vi "Sandbox.vi"() -> ()   [LabVIEW 2019, in "SV_Publisher.lvclass"]
uses:
  SV_Publisher.lvclass
  TypeDef/Needle Valve Data.ctl
  modbus engine custom/MB_ENGINE_class/Engine State.ctl
  TypeDef/Needle Valve State.ctl
  modbus engine custom/MB_ENGINE_class/Engine Alarms.ctl
  modbus engine custom/MB_ENGINE_class/Settings.ctl
  modbus engine custom/MB_ENGINE_class/Limits Status.ctl
  SV_Publisher.lvclass/SV_Publisher.ctl
  Set SV.vi/1ae5d02c-efd0-450a-8aa4-8388e25d05bc.vi
  modbus engine custom/MB_ENGINE_class/MB_ENGINE.lvclass
panel:
  in  "?":T1={"Engine State"=8, "StateValveModbus"=enum."IDLE", "Alarms"={"OL"=FALSE, "TF"=FALSE, "STL"=FALSE, "OCP"=FALSE, "CPUV"=FALSE, "UVLO"=FALSE, "SPI_ERROR"=FALSE, "Fault"=FALSE, "OL 2"=FALSE, "TF 2"=FALSE, "STL 2"=FALSE, "OCP 2"=FALSE, "CPUV 2"=FALSE, "UVLO 2"=FALSE, "reserved"=TRUE, "InitDone"=TRUE}, "RAW Possition"=124110, "Angele"=0.0, "Step"=0, "Encoder"=0, "Kinematic"={"ACC Steps Per Sec^2"=100, "DEC Steps Per Sec^2"=100, "Min Velosity Step Per Sec"=100, "Max Velosity Step Per Sec"=200, "MicroStep"=16}, "Limits"={"Fault 2 Switch"=FALSE, "Fault 1 Switch"=FALSE, "Center(Home)"=FALSE, "Lower Limit"=FALSE, "Upper Limit"=FALSE}} {"Engine State" items=["ACCELERATING", "DECELERATINGTOSTOP", "DECELERATING", "STEADY", "INDEX_ACCEL", "NDEX_RUN", "INDEX_DECEL", "INDEX_DWELL", "INACTIVE", "STANDBY", "STANDBYTOINACTIVE"]}
  in  "set 2":bool
  in  "set 1":bool
  in  "stop":bool
  out "error out":errorcluster
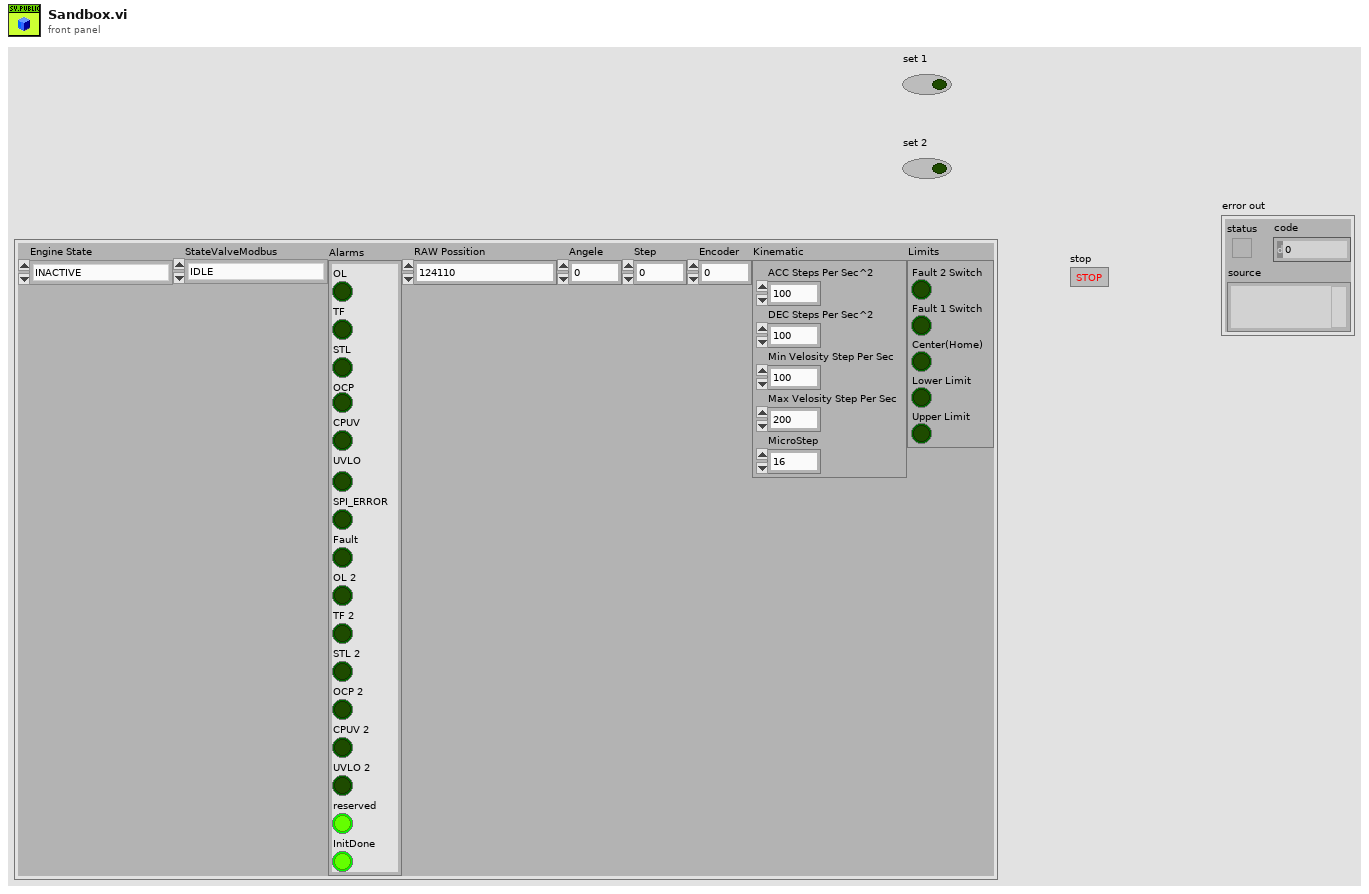
[diagram p1: front panel]
types:
  T1 = typedef "Needle Valve Data.ctl" = cluster{"Engine State":T2, "StateValveModbus":T3, "Alarms":T4, "RAW Possition":i32, "Angele":dbl, "Step":i32, "Encoder":i32, "Kinematic":T5, "Limits":T6}
  T2 = typedef "MB_ENGINE.lvclass/Engine State.ctl" = u16
  T3 = typedef "Needle Valve State.ctl" = enum16{"IDLE", "OPENING", "CLOSING", "STOP"}
  T4 = typedef "MB_ENGINE.lvclass/Engine Alarms.ctl" = cluster{"OL":bool, "TF":bool, "STL":bool, "OCP":bool, "CPUV":bool, "UVLO":bool, "SPI_ERROR":bool, "Fault":bool, "OL 2":bool, "TF 2":bool, "STL 2":bool, "OCP 2":bool, "CPUV 2":bool, "UVLO 2":bool, "reserved":bool, "InitDone":bool}
  T5 = typedef "MB_ENGINE.lvclass/Settings.ctl" = cluster{"ACC Steps Per Sec^2":u16, "DEC Steps Per Sec^2":u16, "Min Velosity Step Per Sec":u16, "Max Velosity Step Per Sec":u16, "MicroStep":u16}
  T6 = typedef "MB_ENGINE.lvclass/Limits Status.ctl" = cluster{"Fault 2 Switch":bool, "Fault 1 Switch":bool, "Center(Home)":bool, "Lower Limit":bool, "Upper Limit":bool}
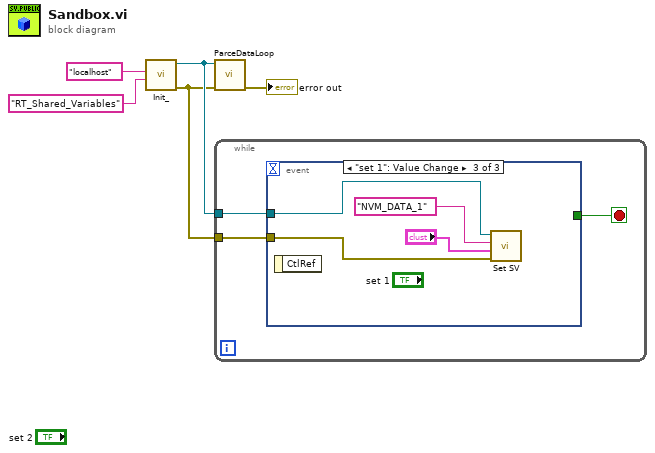
[diagram p0: block diagram]
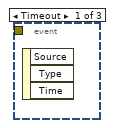
[diagram p2: hidden frame]
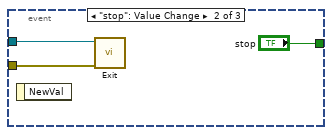
[diagram p3: hidden frame]
diagram:
  n1 = call "Init_.vi"("lib"="RT_Shared_Variables", "host"="localhost") -> ("error out"=w2:errorcluster, "SV_Publisher out"=w3:refnum<class "SV_Publisher.lvclass">)  [unwired: 8 in]
  n2 = call "ParceDataLoop.vi"("error in (no error)"=w2, "SV_Publisher in"=w3) -> ("error out"=→"error out":errorcluster)  [unwired: 9 in]
  n3 = while {
    tunnel: w3 -> [w7]
    tunnel: w2 -> [w6]
    stop <- w8 stop-if-true
    n4 = event shown="[2] \"set 1\": Value Change" {
      selector: _ -> [_ _ _]
      dyn-events: _ -> [_ _ _]
      timeout: _ -> [_ _ _]
      tunnel: [_ "stop" _] -> w8
      tunnel: w7 -> [_ w10 w15]
      tunnel: w6 -> [_ w9 w14]
      event Timeout {
        n5 = event-data() -> ()  [unwired: 1 in, 3 out]
      }
      event "stop": Value Change {
        n6 = event-data() -> ()  [unwired: 1 in, 1 out]
        n7 = call "Exit.vi"("error in (no error)"=w9, "SV_Publisher in"=w10) -> ()  [unwired: 8 in, 2 out]
      }
      event "set 1": Value Change {
        n8 = event-data() -> ()  [unwired: 1 in, 1 out]
        n9 = call "Set SV.vi"("error in (no error)"=w14, "SV Value"="?", "SV Name"="NVM_DATA_1", "SV_Publisher in"=w15) -> ()  [unwired: 6 in, 2 out]
      }
    }
  }
